vi "Write Element of TagDistanceArray.vi"(8 "error in (no error)":errorcluster, 9 "TagDistance":T1={"Tag.lvclass"=refnum, "Distance"=-1.0}, 11 "Anchor in":refnum<class "Anchor.lvclass">) -> (0 "error out":errorcluster, 3 "Anchor out":refnum<class "Anchor.lvclass">)   [LabVIEW 2014, in "Anchor.lvclass"]
uses:
  Anchor.lvclass
  Tag.lvclass
  Anchor.lvclass/Anchor.ctl
panel:
  out "index":i32
  out "has element?":bool
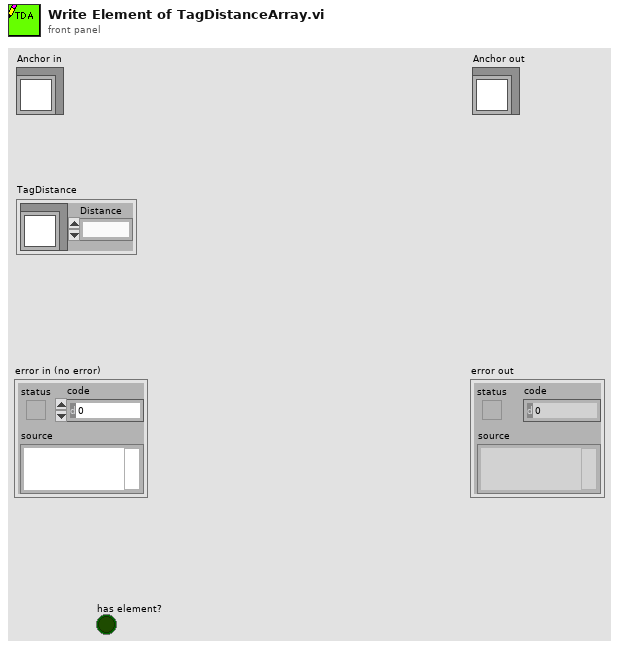
[diagram p1: front panel]
types:
  T1 = cluster{"Tag.lvclass":refnum<class "Tag.lvclass">, "Distance":dbl}
  T2 = cluster{"Tag.lvclass":refnum<class "Tag.lvclass">, "Distance":dbl}[]
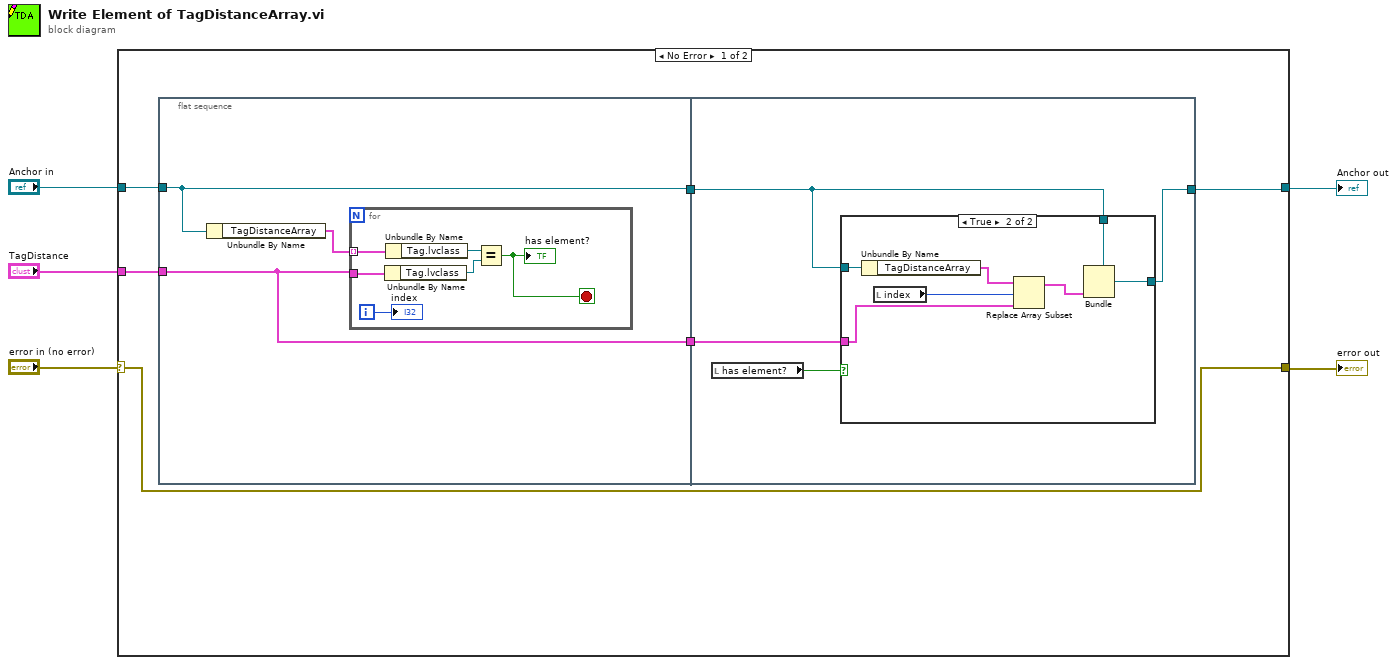
[diagram p0: block diagram]
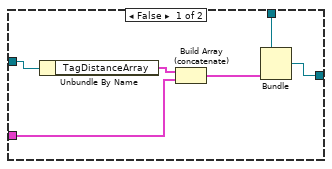
[diagram p2: hidden frame]
diagram:
  n1 = case shown="No Error" "error in (no error)" {
    selector: "error in (no error)" -> [w11 w38]
    tunnel: [w11 w38] -> w4
    tunnel: [w6 w39] -> w2
    tunnel: "Anchor in" -> [w9 w39]
    tunnel: "TagDistance" -> [w10 _]
    frame No Error {
      n2 = flat-sequence {
        tunnel: w10 -> [w12]
        tunnel: w9 -> [w13]
        tunnel: [w13] -> w8
        tunnel: [w12] -> w7
        tunnel: [w21] -> w6
        tunnel: w8 -> [w22]
        tunnel: w7 -> [w23]
        frame #0 {
          n3 = Unbundle By Name(w13) -> ("TagDistanceArray"=w14:T2)
          n4 = for {
            tunnel: w14 -> [w20] mode=indexing
            tunnel: w12 -> [w19]
            i -> [w15]
            stop <- w16 stop-if-true
            n5 = Unbundle By Name(w19) -> ("Tag.lvclass"=w18:refnum<class "Tag.lvclass">)
            n6 = Unbundle By Name(w20) -> ("Tag.lvclass"=w17:refnum<class "Tag.lvclass">)
            n7 = Equal?(x=w17, y=w18) -> (x = y?=w16:bool)
            "has element?" <- w16
            "index" <- w15
          }
        }
        frame #1 {
          n8 = local read "has element?"() -> (w24:bool)
          n9 = case shown="True" w24 {
            tunnel: w22 -> [w30 w37]
            tunnel: w23 -> [w28 w32]
            tunnel: w22 -> [w27 w35]
            tunnel: [w25 w33] -> w21
            frame False {
              n10 = Unbundle By Name(w30) -> ("TagDistanceArray"=w29:T2)
              n11 = Build Array (concatenate)(w29, w28) -> (w26:T2)
              n12 = Bundle(cluster=w27, w26) -> (w25:refnum<class "Anchor.lvclass">)  [unwired: 3 in]
            }
            frame True {
              n13 = Unbundle By Name(w37) -> ("TagDistanceArray"=w36:T2)
              n14 = local read "index"() -> (w31:i32)
              n15 = Replace Array Subset(array=w36, new element=w32, index=w31) -> (w34:T2)
              n16 = Bundle(cluster=w35, w34) -> (w33:refnum<class "Anchor.lvclass">)  [unwired: 3 in]
            }
          }
        }
      }
    }
    frame Error {
    }
  }
  "error out" <- w4
  "Anchor out" <- w2
